vi "PH_Beckhoff.set failure values.vi"(0 "i ref in":refnum<vi>, 5 "error in":errorcluster) -> (11 "Failure Values Digital Outputs":bool[](array[boolean]), 13 "Failure Values Digital Inputs":bool[](array[boolean]), 14 "i ref out":refnum<vi>, 15 "Failure Values Sonderklemmen Inputs":u32[](array[numeric]), 16 "Failure Values Analog Inputs":u32[](array[numeric]), 17 "Failure Values Analog Outputs":u32[](array[numeric]), 18 "Read and write successful?":bool, 19 "error out":errorcluster)   [LabVIEW 2014, in "PH_Beckhoff.lvlib"]
doc: "This VI sets neutral values (0 or false) to all Beckhoff values, for example to be used in case of a failure. Read successful is set to false."
uses:
  PH_Beckhoff.lvlib
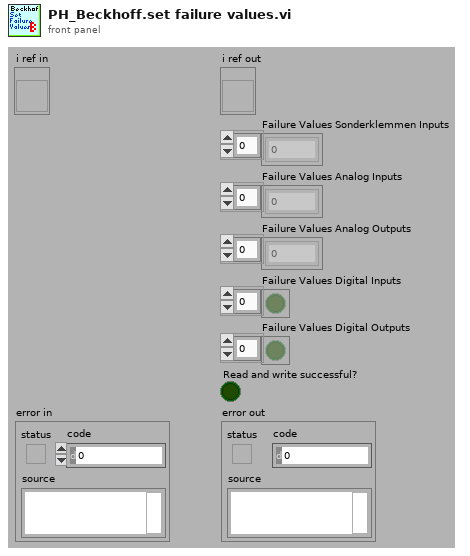
[diagram p1: front panel]
types:
  T1 = typedef "PH_Beckhoff.lvlib/PH_Beckhoff.i attribute.ctl" = cluster{"GUI Refs":T2, "operation?":bool, "Default Prdc Interval":i32, "Connection":T3, "AMS Net ID":T4, "Klemmencluster: # of":T5, "Values":T6, "IP":string, "Description":string, "configured?":bool, "Change Manager":cluster{"Detemination wanted?":bool, "Values changed at":cluster{"Sonderklemmen Inputs":i32[], "Analog Inputs":i32[], "Analog Outputs":i32[], "Digital Inputs":i32[], "Digital Outputs":i32[]}}, "Difference to handle an analog input as change":u32}
  T2 = typedef "PH_Beckhoff.lvlib/PH_Beckhoff.GUI Refs.ctl" = cluster{"ADS Error":refnum<vi>, "Values":refnum<vi>, "configured?":refnum<vi>, "Connection":refnum<vi>, "IP":refnum<vi>, "Prdc Int [ms]":refnum<vi>}
  T3 = typedef "PH_Beckhoff.lvlib/PH_Beckhoff.Connectivity.ctl" = cluster{"DLL?":bool, "Port?":bool, "Client?":bool, "Ping?":bool, "unsuccessful Pings":u32}
  T4 = typedef "Beckhoff - Driver np.lvlib/Beckhoff Access.ctl" = cluster{"DLL path":path, "AMS Net ID":cluster{"1st # of IP":u8, "2nd # of IP":u8, "3rd # of IP":u8, "4th # of IP":u8, "In Port":u8, "Out Port":u8}}
  T5 = typedef "Beckhoff - Driver np.lvlib/Klemmendeclarer.ctl" = cluster{"Offset due to Sonderklemms":u32, "analog Inputs":u32, "analog Outputs":u32, "digital Input Bits":u32, "digital Output Bits":u32}
  T6 = typedef "PH_Beckhoff.lvlib/PH_Beckhoff.Values.ctl" = cluster{"Sonderklemmen Inputs":T7, "Analog Inputs":T8, "Analog Outputs":T10, "Digital Inputs":T11, "Digital Outputs":T12}
  T7 = typedef "PH_Beckhoff.lvlib/PH_Beckhoff.Sonderklemmen Inputs.ctl" = cluster{"Total Length":u32, "Name":string, "Value":u64, "Quality":bool, "Service ID":i32, "Offset":u32, "Length":u32}[]
  T8 = typedef "PH_Beckhoff.lvlib/PH_Beckhoff.Analog Inputs.ctl" = cluster{"Name":string, "Value":u32, "Quality":bool, "Service ID":i32, "Sca Type":T9}[]
  T9 = typedef "PH_Beckhoff.lvlib/PH_Beckhoff.Scaling Type.ctl" = enum16{"none", "0 ... 15 Bit -> 0 ... 5", "0 ... 15 Bit -> 0 ... 10", "0 ... 15 Bit -> 0 ... 25", "0 ... 15 Bit -> 4 ... 20", "0 ... 15 Bit -> 0 ... 1", "0 ... 15 Bit -> 0 ... 20000", "0 ... 15 Bit -> 0 ... 24000"}
  T10 = typedef "PH_Beckhoff.lvlib/PH_Beckhoff.Analog Outputs.ctl" = cluster{"Name":string, "Value":u32, "Quality":bool, "Wanted Value":u32, "Service ID":i32, "Sca Type":T9}[]
  T11 = typedef "PH_Beckhoff.lvlib/PH_Beckhoff.Digital Inputs.ctl" = cluster{"Name":string, "Value":bool, "Quality":bool, "Service ID":i32, "inverted?":bool}[]
  T12 = typedef "PH_Beckhoff.lvlib/PH_Beckhoff.Digital Outputs.ctl" = cluster{"Name":string, "Value":bool, "Quality":bool, "Wanted Value":bool, "Service ID":i32, "inverted?":bool}[]
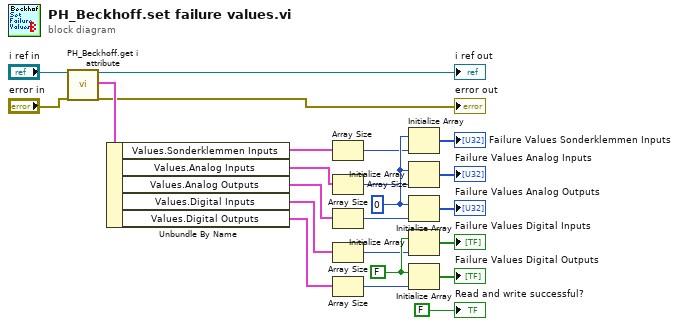
[diagram p0: block diagram]
diagram:
  w13 = u32 0 ("Boolean array[0]")
  w5 = FALSE ("read successful?")
  n1 = call "PH_Beckhoff.get i attribute.vi"("i ref in"="i ref in", "error in (no error)"="error in") -> ("i ref out"=→"i ref out":refnum<vi>, "i attribute"=w18:T1, "error out"=→"error out":errorcluster)  [unwired: 15 in]
  n2 = Unbundle By Name(w18) -> ("Values.Sonderklemmen Inputs"=w19:T7, "Values.Analog Inputs"=w20:T8, "Values.Analog Outputs"=w21:T10, "Values.Digital Inputs"=w22:T11, "Values.Digital Outputs"=w23:T12)
  n3 = Array Size(array=w19) -> (size(s)=w11:i32)
  n4 = Array Size(array=w20) -> (size(s)=w7:i32)
  n5 = Array Size(array=w21) -> (size(s)=w9:i32)
  n6 = Array Size(array=w22) -> (size(s)=w4:i32)
  n7 = Array Size(array=w23) -> (size(s)=w2:i32)
  n8 = Initialize Array(w13, w11) -> (→"Failure Values Sonderklemmen Inputs":u32[])
  n9 = Initialize Array(w13, w7) -> (→"Failure Values Analog Inputs":u32[])
  n10 = Initialize Array(w13, w9) -> (→"Failure Values Analog Outputs":u32[])
  n11 = Initialize Array(w5, w4) -> (→"Failure Values Digital Inputs":bool[])
  n12 = Initialize Array(w5, w2) -> (→"Failure Values Digital Outputs":bool[])
  "Read and write successful?" <- FALSE ("read successful?")
